vi "Set Delimiter.vi"(8 "error in (no error)":errorcluster, 10 "Namespace Delimiter":string(combo)=":") -> (0 "error out":errorcluster)   [LabVIEW 2020, in "Tag Engine Core.lvlib" / "Tag Core.lvclass"]
doc: "_SubVI_"
uses:
  Tag Core.lvclass
  Tag Core.lvclass/Tag Core.ctl
panel:
  # "Default delimiter is \":'\nBut you could use \"::\"\nor \"_\""
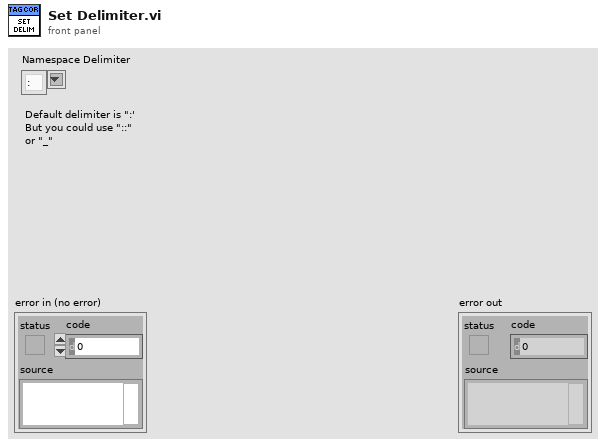
[diagram p1: front panel]
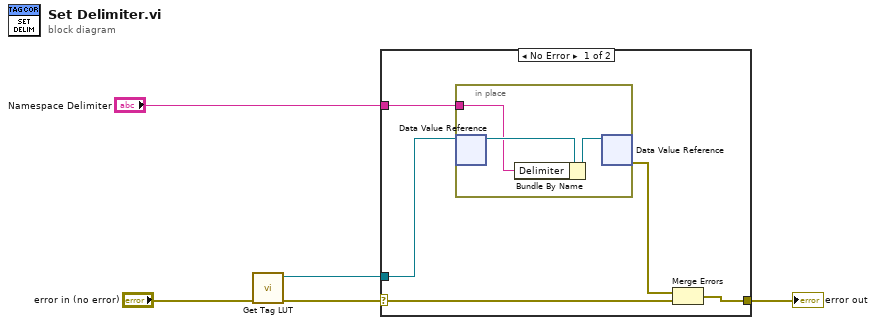
[diagram p0: block diagram]
diagram:
  n1 = call "Get Tag LUT.vi"("error in (no error)"="error in (no error)") -> ("error out"=w3:errorcluster, "Tag LUT Out"=w2:refnum<data-value>)  [unwired: 9 in]
  n2 = case shown="No Error" w3 {
    selector: w3 -> [w8 w14]
    tunnel: [w7 w14] -> w5
    tunnel: w2 -> [w10 _]
    tunnel: "Namespace Delimiter" -> [w9 _]
    frame No Error {
      n3 = in-place {
        in-place-border: w9 -> [w11]
        n4 = in-place-dvr #1(w10) -> (w13:refnum<class "Tag Core.lvclass">)  [unwired: 1 out]
        n5 = Bundle By Name(cluster=w13, "Delimiter"=w11) -> (w12:refnum<class "Tag Core.lvclass">)
        n6 = in-place-dvr #1(w12) -> (w6:errorcluster)  [unwired: 1 out]
      }
      n7 = Merge Errors(w6, w8) -> (w7:errorcluster)
    }
    frame Error {
    }
  }
  "error out" <- w5
